vi "IVI_h5.vi"(3 "Model":string, 4 "TYPE":string="CH_A#", 5 "Manufacturer":string, 6 "Bin size":i16=1, 7 "SQUID":string="    6", 8 "error in":errorcluster, 9 "Waveform Data":waveform(dbl)[](graph)=[{"t0"=timestamp(1.3199999999947629e-08 s since 1904-01-01), "dt"=1e-06, "Y"=array[1000 elements]}, {"t0"=timestamp(1.3199999999947629e-08 s since 1904-01-01), "dt"=1e-06, "Y"=array[1000 elements]}], 10 "Channels":T1[](array[typedef])=[{"channel name"="CHANNEL1", "probe attenuation"=1.0, "vertical offset"=0.0, "vertical range"=6.0, "vertical coupling"=1, "input impedance"=1000000.0}, {"channel name"="CHANNEL2", "probe attenuation"=1.0, "vertical offset"=0.0, "vertical range"=1.0, "vertical coupling"=1, "input impedance"=1000000.0}] {"input impedance" format="%#_13g"; "vertical coupling" items=["AC", "DC", "GND"]; "vertical range" format="%.3f"; "vertical offset" format="%.3f"; "probe attenuation" format="%.3f"}, 11 "H5":path[](array[path])=[path "D:/Data/2015/08/19/20150819_115740/20150819_115740.h5"]) -> (0 "error out":errorcluster)   [LabVIEW 2013]
uses:
  Acquisition/IVI_chan.ctl
panel:
  out "t0":dbl
  out "Attributes":variant=variant("dt"=variant(dbl 1e-06), "vertical coupling"=variant(string "DC"))
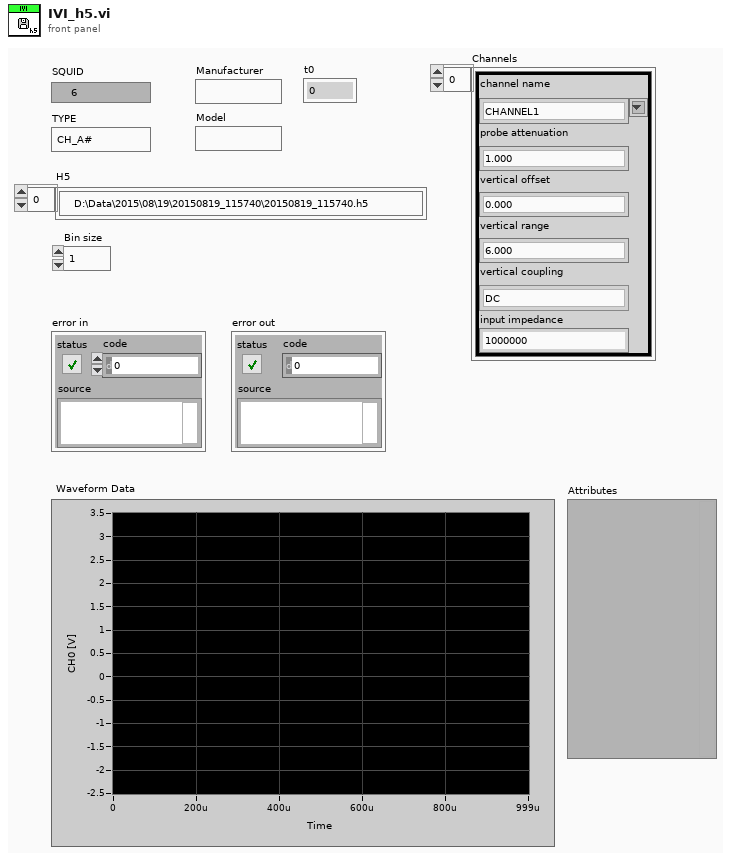
[diagram p1: front panel]
types:
  T1 = typedef "IVI_chan.ctl" = cluster{"channel name":string, "probe attenuation":dbl, "vertical offset":dbl, "vertical range":dbl, "vertical coupling":i32, "input impedance":dbl}
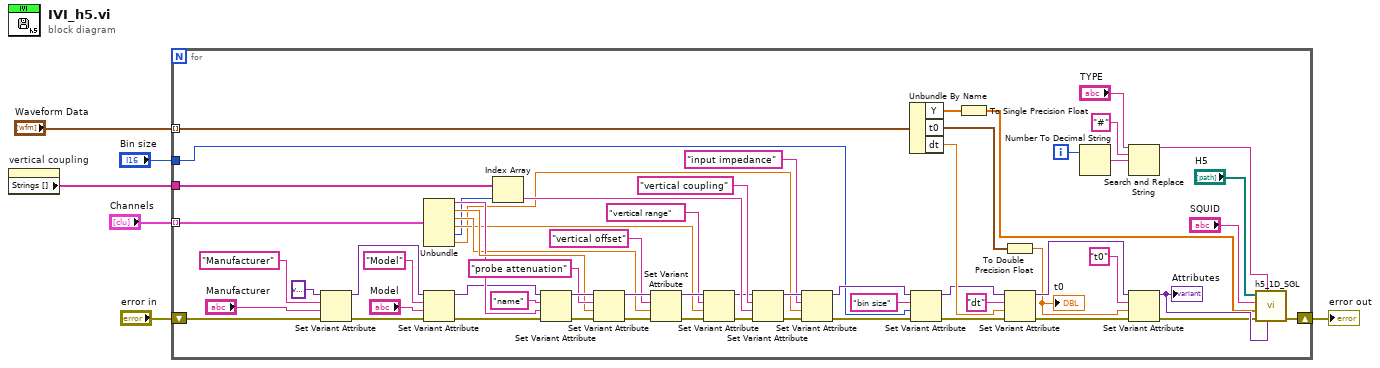
[diagram p0: block diagram]
diagram:
  n1 = property on="vertical coupling" class="Ring (strict)"() -> ("Strings []"=w2:string[])  [unwired: 2 in, 2 out]
  n2 = for {
    tunnel: "Channels" -> [w53] mode=indexing
    shift-right: [w55] -> w5
    shift-left: "error in" -> [w20]
    tunnel: w2 -> [w60]
    tunnel: "Waveform Data" -> [w63] mode=indexing
    tunnel: "Bin size" -> [w7]
    i -> [w67]
    n3 = Set Variant Attribute(Variant=variant ("variant"), name="Manufacturer", value="Manufacturer", error in=w20) -> (Variant out=w27:variant, error out=w22:errorcluster)  [unwired: 1 out]
    n4 = Unbundle(w53) -> ("channel name"=w41:string, "probe attenuation"=w42:dbl, "vertical offset"=w40:dbl, "vertical range"=w39:dbl, "vertical coupling"=w38:i32, "input impedance"=w13:dbl)
    n5 = Set Variant Attribute(Variant=w27, name="Model", value="Model", error in=w22) -> (Variant out=w26:variant, error out=w21:errorcluster)  [unwired: 1 out]
    n6 = Index Array(array=w60, index=w38) -> (element=w57:string)
    n7 = Set Variant Attribute(Variant=w26, name="name", value=w41, error in=w21) -> (Variant out=w52:variant, error out=w44:errorcluster)  [unwired: 1 out]
    n8 = Set Variant Attribute(Variant=w52, name="probe attenuation", value=w42, error in=w44) -> (Variant out=w51:variant, error out=w43:errorcluster)  [unwired: 1 out]
    n9 = Set Variant Attribute(Variant=w51, name="vertical offset", value=w40, error in=w43) -> (Variant out=w50:variant, error out=w45:errorcluster)  [unwired: 1 out]
    n10 = Set Variant Attribute(Variant=w50, name="vertical range", value=w39, error in=w45) -> (Variant out=w37:variant, error out=w36:errorcluster)  [unwired: 1 out]
    n11 = Set Variant Attribute(Variant=w37, name="vertical coupling", value=w57, error in=w36) -> (Variant out=w15:variant, error out=w16:errorcluster)  [unwired: 1 out]
    n12 = Set Variant Attribute(Variant=w15, name="input impedance", value=w13, error in=w16) -> (Variant out=w12:variant, error out=w10:errorcluster)  [unwired: 1 out]
    n13 = Unbundle By Name(w63) -> ("Y"=w18:dbl[], "t0"=w35:timestamp, "dt"=w58:dbl)
    n14 = Set Variant Attribute(Variant=w12, name="bin size", value=w7, error in=w10) -> (Variant out=w11:variant, error out=w9:errorcluster)  [unwired: 1 out]
    n15 = To Single Precision Float(number=w18) -> (single precision float=w17:sgl[])
    n16 = To Double Precision Float(number=w35) -> (double precision float=w29:dbl)
    "t0" <- w29
    n17 = Set Variant Attribute(Variant=w11, name="dt", value=w58, error in=w9) -> (Variant out=w33:variant, error out=w31:errorcluster)  [unwired: 1 out]
    n18 = Number To Decimal String(number=w67) -> (decimal integer string=w64:string)  [unwired: 1 in]
    n19 = Search and Replace String(input string="TYPE", search string="#", replace string=w64) -> (result string=w61:string)  [unwired: 5 in, 3 out]
    n20 = Set Variant Attribute(Variant=w33, name="t0", value=w29, error in=w31) -> (Variant out=w34:variant, error out=w32:errorcluster)  [unwired: 1 out]
    "Attributes" <- w34
    n21 = call "h5_1D_SGL.vi"("Attributes"=w34, "TYPE"=w61, "error in (no error)"=w32, "1D SGL"=w17, "SQUID"="SQUID", "H5"="H5") -> ("error out"=w55:errorcluster)  [unwired: 4 in, 1 out]
  }
  "error out" <- w5
